vi "变矩器及前轮左右温度标定.vi"(11 "变矩器，前轮左和右信号输入":dbl) -> (3 "变矩器，前轮左和右信号输出":dbl)   [LabVIEW 2016]
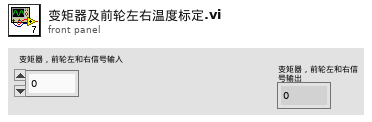
[diagram p1: front panel]
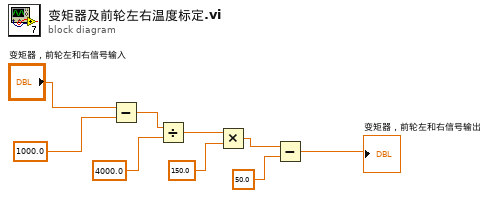
[diagram p0: block diagram]
diagram:
  n1 = Subtract(x="变矩器，前轮左和右信号输入", y=1000.0) -> (x-y=w7:dbl)
  n2 = Divide(x=w7, y=4000.0) -> (x/y=w5:dbl)
  n3 = Multiply(x=w5, y=150.0) -> (x*y=w3:dbl)
  n4 = Subtract(x=w3, y=50.0) -> (x-y=→"变矩器，前轮左和右信号输出":dbl)
